vi "Replace EmptyCell Mark.vi"(8 "error in (no error)":errorcluster, 9 "EmptyCellToken(^[\\/]$)":string="^[\\/]$", 11 "CfgTable in":string[][](array[string])) -> (0 "error out":errorcluster, 3 "CfgTable out":string[][](array[string]))   [LabVIEW 2017, in "ClusterCfgTable.lvlib"]
doc: "Replaces the empty-cell marker in a configuration table with an empty string. The marker is given by EmptyCellToken and defaults to ^[\\/]$."
uses:
  ClusterCfgTable.lvlib
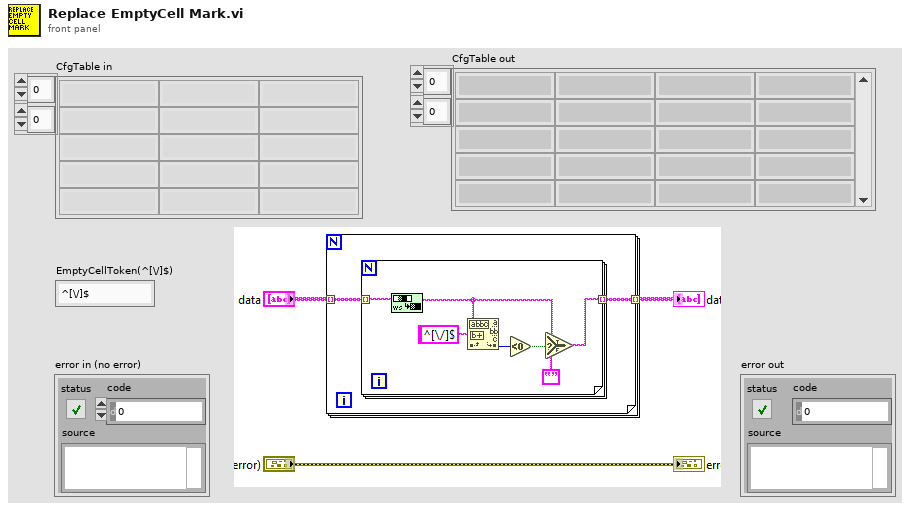
[diagram p1: front panel]
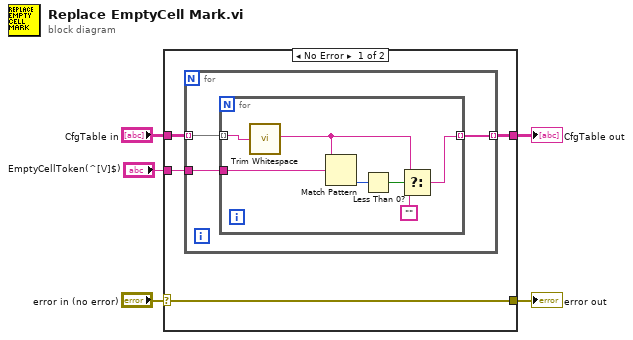
[diagram p0: block diagram]
diagram:
  n1 = case shown="No Error" "error in (no error)" {
    selector: "error in (no error)" -> [w6 w21]
    tunnel: [w9 w20] -> w5
    tunnel: "CfgTable in" -> [w8 w20]
    tunnel: "EmptyCellToken(^[\\/]$)" -> [w7 _]
    tunnel: [w6 w21] -> w2
    frame No Error {
      n2 = for {
        tunnel: w8 -> [w11] mode=indexing
        tunnel: [w12] -> w9 mode=indexing
        tunnel: w7 -> [w10]
        n3 = for {
          tunnel: [w14] -> w12 mode=indexing
          tunnel: w11 -> [w19] mode=indexing
          tunnel: w10 -> [w13]
          n4 = call <vilib>:"Trim Whitespace.vi"("string"=w19) -> ("trimmed string"=w16:string)  [unwired: 1 in]
          n5 = Match Pattern(string=w16, regular expression=w13) -> (offset past match=w18:i32)  [unwired: 1 in, 3 out]
          n6 = Less Than 0?(x=w18) -> (x < 0?=w17:bool)
          n7 = Select(t=w16, s=w17, f="") -> (s? t:f=w14:string)
        }
      }
    }
    frame Error {
    }
  }
  "error out" <- w2
  "CfgTable out" <- w5
